vi "Pixel integration - Line begin and pixel duration.vi"(6 "pixel period (ps)":i64, 7 "line_begin_ch":i32, 8 "error in (no error)":errorcluster, 9 "pixel integration, (ps)":i64=1000, 10 "pixels in line":i32, 11 "tagger in":refnum<k24>) -> (0 "error out":errorcluster, 1 "pixel_end_ch":i32, 2 "pixel_start_ch":i32, 3 "event generator refs":T1)   [LabVIEW 2014]
uses:
  SwabianInstruments.TimeTagger
  <vilib>/ErrorRing/Error Ring.xnode
  <vilib>/Utility/error.llb/Error Cluster From Error Code.vi
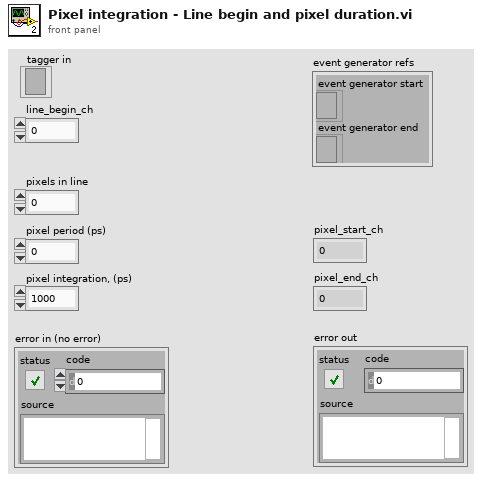
[diagram p1: front panel]
types:
  T1 = cluster{"event generator start":refnum<k24>, "event generator end":refnum<k24>}
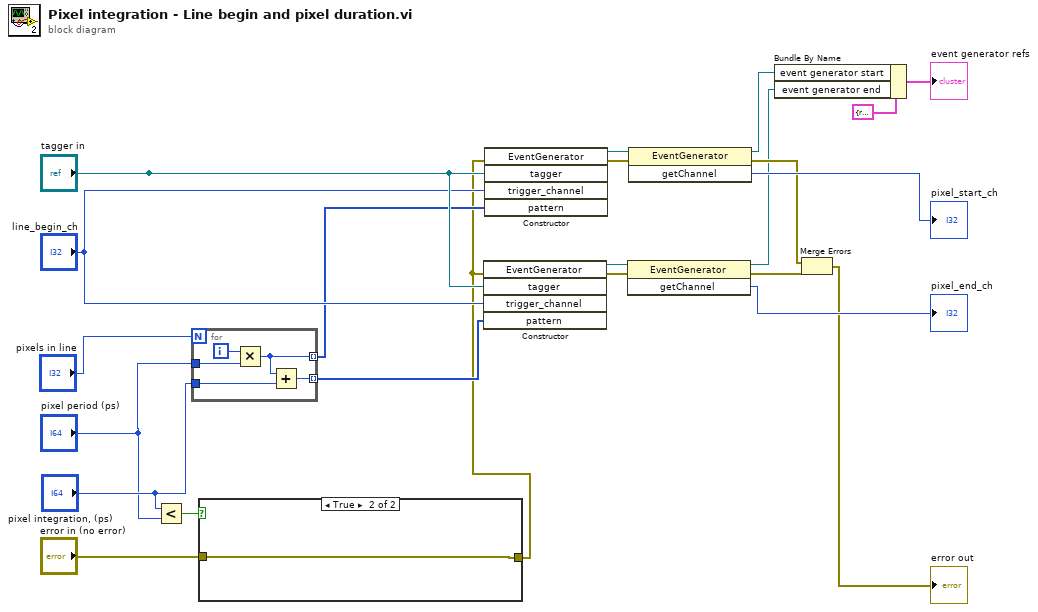
[diagram p0: block diagram]
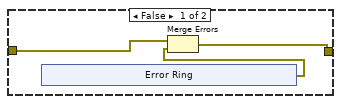
[diagram p2: hidden frame]
diagram:
  n1 = Less?(x="pixel integration, (ps)", y="pixel period (ps)") -> (x < y?=w7:bool)
  n2 = for {
    N: "pixels in line" -> [_]
    tunnel: "pixel period (ps)" -> [w26]
    tunnel: [w28] -> w10 mode=indexing
    tunnel: "pixel integration, (ps)" -> [w27]
    tunnel: [w24] -> w11 mode=indexing
    i -> [w25]
    n3 = Multiply(x=w25, y=w26) -> (x*y=w28:i64)
    n4 = Add(x=w28, y=w27) -> (x+y=w24:i64)
  }
  n5 = case shown="True" w7 {
    tunnel: "error in (no error)" -> [w31 w37]
    tunnel: [w29 w37] -> w8
    frame False {
      n6 = xnode "Error Ring"() -> ("error out"=w30:errorcluster)
      n7 = Merge Errors(w31, w30) -> (w29:errorcluster)
    }
    frame True {
    }
  }
  n8 = constructor class="EventGenerator"(error in=w8, "tagger"="tagger in", "trigger_channel"="line_begin_ch", "pattern"=w11) -> (reference out=w19:refnum<k24>, error out=w20:errorcluster)  [unwired: 2 in, 4 out]
  n9 = constructor class="EventGenerator"(error in=w8, "tagger"="tagger in", "trigger_channel"="line_begin_ch", "pattern"=w10) -> (reference out=w22:refnum<k24>, error out=w23:errorcluster)  [unwired: 2 in, 4 out]
  n10 = invoke class="EventGenerator" method="getChannel"(reference=w19, error in=w20) -> (reference out=w3:refnum<k24>, error out=w14:errorcluster, "getChannel"=→"pixel_end_ch":i32)  [unwired: 1 in]
  n11 = invoke class="EventGenerator" method="getChannel"(reference=w22, error in=w23) -> (reference out=w4:refnum<k24>, error out=w13:errorcluster, "getChannel"=→"pixel_start_ch":i32)  [unwired: 1 in]
  n12 = Bundle By Name(cluster=T1 {"event generator start"=refnum, "event generator end"=refnum} ("input cluster"), "event generator start"=w4, "event generator end"=w3) -> (→"event generator refs":T1)
  n13 = Merge Errors(w13, w14) -> (→"error out":errorcluster)
